vi "Render Ship.vi"(7 "Renderer":refnum<class "Renderer.lvclass">, 8 "error in (no error)":errorcluster, 10 "Camera":refnum<class "Camera.lvclass">, 11 "Ship in":refnum<class "Ship.lvclass">) -> (0 "error out":errorcluster)   [LabVIEW 2021, in "Ship.lvclass"]
uses:
  Ship.lvclass
  C:/dev/LabVIEW/LabMelee/Source/Application Specific/Element/Element.lvclass
  Camera/Camera.lvclass
  Renderer/Renderer.lvclass
  Element/Element.lvclass/Element.ctl
  Motion/Motion.lvclass/Motion.ctl
  Ship.lvclass/Ship.ctl
  Camera/Camera.lvclass/Camera.ctl
  Vector 2D/Vector 2D.lvclass/Vector 2D.ctl
  Renderer/Renderer.lvclass/Renderer.ctl
  Texture/Texture.lvclass/Texture.ctl
  Motion/Motion.lvclass
  Element/Element.lvclass
  Resource Manager/Resource Manager.lvclass
  Vector 2D/Vector 2D.lvclass
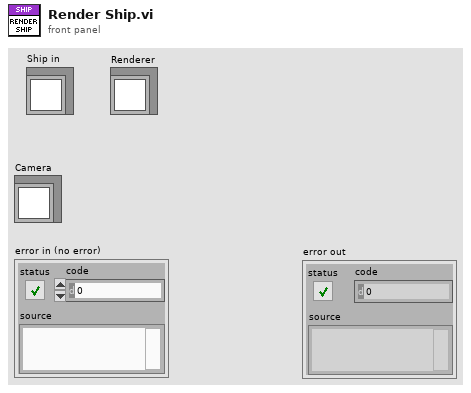
[diagram p1: front panel]
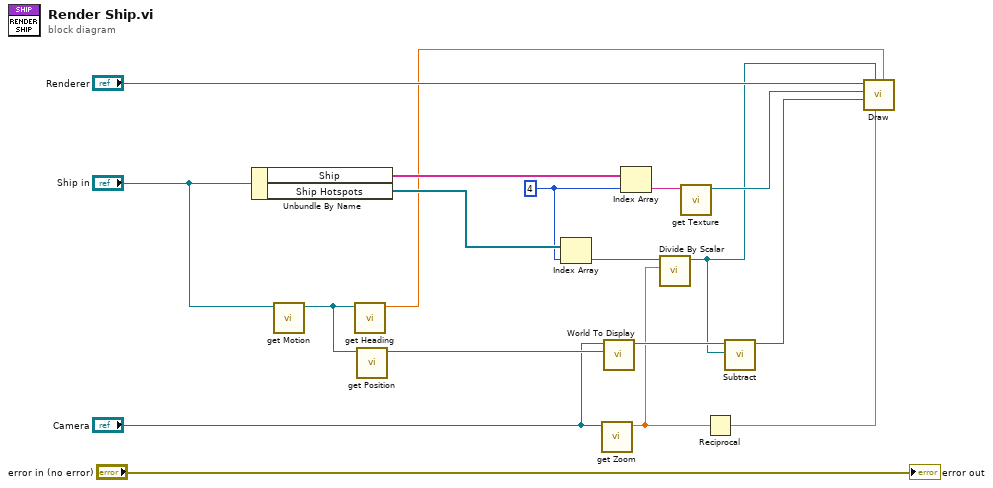
[diagram p0: block diagram]
diagram:
  w3 = 4 ("Texture Index")
  n1 = Unbundle By Name("Ship in") -> ("Ship"=w18:string[], "Ship Hotspots"=w17:refnum<class "Vector 2D.lvclass">[])
  n2 = call "get Motion.vi"("Element in"="Ship in") -> ("Motion"=w15:refnum<class "Motion.lvclass">)  [unwired: 10 in]
  n3 = call "get Heading.vi"("Motion in"=w15) -> ("Heading [deg]"=w2:sgl)  [unwired: 10 in]
  n4 = call "get Position.vi"("Motion in"=w15) -> ("Displacement"=w11:refnum<class "Vector 2D.lvclass">)  [unwired: 10 in]
  n5 = Index Array(array=w17, index=w3) -> (element=w6:refnum<class "Vector 2D.lvclass">)
  n6 = call "get Zoom.vi"("Camera in"="Camera") -> ("Zoom Level"=w5:sgl)  [unwired: 10 in]
  n7 = call "World To Display.vi"("World Position"=w11, "Camera in"="Camera") -> ("Display Position"=w7:refnum<class "Vector 2D.lvclass">)  [unwired: 9 in]
  n8 = Index Array(array=w18, index=w3) -> (element=w14:string)
  n9 = call "Divide By Scalar.vi"("x"=w5, "A"=w6) -> ("Ax"=w1:refnum<class "Vector 2D.lvclass">)  [unwired: 9 in]
  n10 = call "get Texture.vi"("Texture Name"=w14) -> ("Texture"=w8:refnum<class "Texture.lvclass">)  [unwired: 10 in]
  n11 = Reciprocal(x=w5) -> (1/x=w9:sgl)
  n12 = call "Subtract.vi"("B"=w1, "A"=w7) -> ("A-B"=w4:refnum<class "Vector 2D.lvclass">)  [unwired: 9 in]
  n13 = call "Draw.vi"("Angle"=w2, "Scale"=w9, "Rotation Center"=w1, "Destination"=w4, "Texture"=w8, "Renderer"="Renderer") -> ()  [unwired: 5 in, 1 out]
  "error out" <- "error in (no error)"
